vi "GetInitialValue.vi"(8 "error in":errorcluster, 10 "Channel Number (1-4)":T1=1 items=["Channel 1"=1, "Channel 2"=2, "Channel 3"=3, "Channel 4"=4], 11 "VISA resource name":refnum<visa-resource-name>) -> (0 "error out":errorcluster, 1 "Current interval initial value":sgl, 2 "Current interval initial value string":string, 3 "VISA resource name out":refnum<visa-resource-name>)   [LabVIEW 2023, in "Thermotron 8800.lvlib"]
doc: "IVAL\nCommand name: Send initial value\nCommand type: System status\nDescription: Queries the 8800 for the current interval’s initial value parameter for channel n (1 through 4). The 8800 sends a decimal value for the selected channel.\nSyntax: IVALn?\nWhere n is the channel number (1 through 4).\nData type: Decimal\nQuery example: IVAL3?\n8800 response: 25.00 (The channel 3 initial value for the current interval is 25.00.)"
uses:
  Thermotron 8800.lvlib
  Private/AnalogInputChannelNumber 1-4.ctl
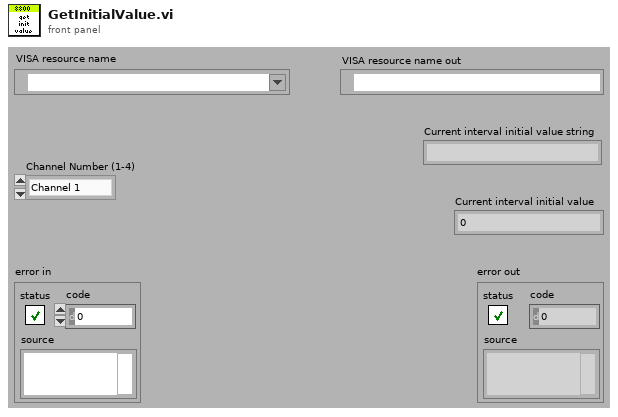
[diagram p1: front panel]
types:
  T1 = typedef "Thermotron 8800.lvlib/AnalogInputChannelNumber 1-4.ctl" = u16
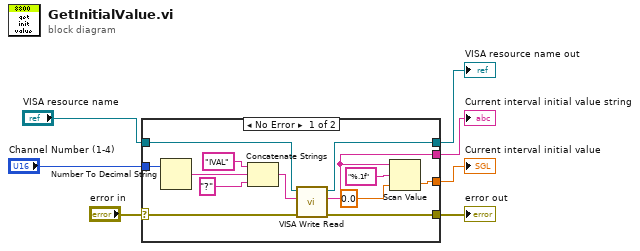
[diagram p0: block diagram]
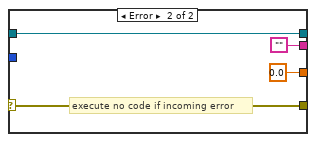
[diagram p2: hidden frame]
diagram:
  n1 = case shown="No Error" "error in" {
    selector: "error in" -> [w19 w24]
    tunnel: [w17 w24] -> w5
    tunnel: [w18 w23] -> w4
    tunnel: "VISA resource name" -> [w15 w23]
    tunnel: "Channel Number (1-4)" -> [w14 _]
    tunnel: [w11 ""] -> w2
    tunnel: [w9 sgl 0.0] -> w1
    frame No Error {
      n2 = Number To Decimal String(number=w14) -> (decimal integer string=w13:string)  [unwired: 1 in]
      n3 = Concatenate Strings("IVAL" ("8800 Command"), w13, "?" ("8800 Command")) -> (w20:string)
      n4 = call "VISA Write Read.vi"("error in (no error)"=w19, "8800 Command"=w20, "VISA Refnum in"=w15) -> ("error out"=w17:errorcluster, "read buffer"=w11:string, "VISA Refnum out"=w18:refnum<visa-resource-name>)  [unwired: 6 in]
      n5 = Scan Value(string=w11, format string="%.1f", default (0 dbl)=sgl 0.0 ("default (0 I32)")) -> (value=w9:sgl)  [unwired: 1 out]
    }
    frame Error {
      # "execute no code if incoming error"
    }
  }
  "VISA resource name out" <- w4
  "error out" <- w5
  "Current interval initial value" <- w1
  "Current interval initial value string" <- w2
